vi "ProcessFCCurrentsSimple.vi"(9 "FC Data":waveform(dbl)[](array[waveform]), 10 "Bouncer Settings":T1 {"LE12C Voltage" format="%_4f"; "LE13C Voltage" format="%_4f"; "14C Voltage" format="%_4f"; "13C Voltage" format="%_4f"; "12C Voltage" format="%_4f"}, 11 "FC Offset":T2={"HE 12C Offset"=0.0, "HE 13CL Offset"=0.0, "HE 13CH Offset"=0.0, "LE FC Scale"=0, "HE C12 Scale"=0, "HE C13 Scale"=18} {"HE C13 Scale" items=["500 mA/V", "200 mA/V", "100 mA/V", "50 mA/V", "20 mA/V", "10 mA/V", "5 mA/V", "2 mA/V", "1 mA/V", "500 uA/V", "200 uA/V", "100 uA/V", "50 uA/V", "20 uA/V", "10 uA/V", "5 uA/V", "2 uA/V", "1 uA/V", "500 nA/V", "200 nA/V", "100 nA/V", "50 nA/V", "20 nA/V", "10 nA/V", "5 nA/V", "2 nA/V", "1 nA/V", "500 pA/V", "200 pA/V", "100 pA/V", "50 pA/V", "20 pA/V", "10 pA/V", "5 pA/V", "2 pA/V", "1 pA/V", ""]; "HE C12 Scale" items=["500 mA/V", "200 mA/V", "100 mA/V", "50 mA/V", "20 mA/V", "10 mA/V", "5 mA/V", "2 mA/V", "1 mA/V", "500 uA/V", "200 uA/V", "100 uA/V", "50 uA/V", "20 uA/V", "10 uA/V", "5 uA/V", "2 uA/V", "1 uA/V", "500 nA/V", "200 nA/V", "100 nA/V", "50 nA/V", "20 nA/V", "10 nA/V", "5 nA/V", "2 nA/V", "1 nA/V", "500 pA/V", "200 pA/V", "100 pA/V", "50 pA/V", "20 pA/V", "10 pA/V", "5 pA/V", "2 pA/V", "1 pA/V", ""]; "LE FC Scale" items=["500 mA/V", "200 mA/V", "100 mA/V", "50 mA/V", "20 mA/V", "10 mA/V", "5 mA/V", "2 mA/V", "1 mA/V", "500 uA/V", "200 uA/V", "100 uA/V", "50 uA/V", "20 uA/V", "10 uA/V", "5 uA/V", "2 uA/V", "1 uA/V", "500 nA/V", "200 nA/V", "100 nA/V", "50 nA/V", "20 nA/V", "10 nA/V", "5 nA/V", "2 nA/V", "1 nA/V", "500 pA/V", "200 pA/V", "100 pA/V", "50 pA/V", "20 pA/V", "10 pA/V", "5 pA/V", "2 pA/V", "1 pA/V", ""]}) -> (1 "Mean Currents":dbl[](array[numeric]), 2 "Output Waveforms":waveform(dbl)[](array[waveform]))   [LabVIEW 2011]
uses:
  FCOffset.ctl
  BouncerParameters.ctl
  <vilib>/Waveform/WDTOps.llb/WDT Get Waveform Subset DBL (LV80).vi
  <vilib>/Analysis/NI_AALBase.lvlib
panel:
  out "Raw":waveform(dbl)[](graph)
  out "HE 13CL":dbl
  out "HE 13CH":waveform(dbl)
  out "LE 13C":dbl
  out "HE 13CH":dbl
  out "LE 12C":dbl
  out "HE 12C":dbl
  out "Bouncer":waveform(dbl)(graph)={"t0"=timestamp(3415120333.4009705 s since 1904-01-01), "dt"=9.999999999999972e-06, "Y"=array[1000 elements], "attributes"=variant("NI_ChannelName"=variant(string "PXI1Slot2/ai0"), "NI_UnitDescription"=variant(string "Volts"))}
  out "LE 13C Cup":waveform(dbl)(graph)={"t0"=timestamp(3415120333.402178 s since 1904-01-01), "dt"=9.999999999999972e-06, "Y"=[0.8050097183722652, 0.24660166407635983, 0.028584441505206795, 0.009584422869030943, 0.009906457076575987, 0.00797425183471986, 0.00797425183471986, 0.007008149216862962, 0.012804764954733521, 0.01312679916455761, 0.010550525492349248, 0.010872559700577551, 0.009584422869030943, 0.01022849128434874, 0.01151662811771772, 0.010872559700577551, 0.010872559700577551, 0.010872559700577551, 0.01022849128434874, 0.009262388661713566, 0.004109841375562904, 0.009262388661713566, 0.01151662811771772, 0.01022849128434874, 0.019567483409006912, 0.01151662811771772, 0.010872559700577551, 0.009906457076575987, 0.009584422869030943, 0.01022849128434874, 0.013448833374609843, 0.01022849128434874, 0.009906457076575987, 0.010550525492349248, 0.00668611501136536, 0.010550525492349248, 0.01022849128434874, 0.01022849128434874, 0.009584422869030943, 0.013448833374609843], "attributes"=variant("NI_ChannelName"=variant(string "PXI1Slot2/ai3"), "NI_UnitDescription"=variant(string "Volts"))}
  out "LE 12C Cup":waveform(dbl)(graph)={"t0"=timestamp(3415120333.4013777 s since 1904-01-01), "dt"=9.999999999999972e-06, "Y"=[0.00668611501136536, 0.007008149216862962, 0.007652217628540168, 0.007330183422587883, 0.00861832024776164, 0.007330183422587883, 0.009262388661713566, 0.01312679916455761, 0.05338107720327494, 0.6781279926088322, 0.8175690797952145, 0.8223996035554544, 0.8240097781590372, 0.8233657083165931, 0.8249758829252316, 0.8230436733958766, 0.8243318130807649, 0.8236877432376466, 0.8243318130807649, 0.8243318130807649, 0.8233657083165931, 0.8278741972420289, 0.8236877432376466, 0.8240097781590372, 0.8227216384754971, 0.8246538480028296, 0.8246538480028296, 0.8246538480028296, 0.8249758829252316, 0.8252979178479707, 0.8214334987973474, 0.8236877432376466, 0.8246538480028296, 0.8246538480028296, 0.8227216384754971, 0.8236877432376466, 0.8243318130807649, 0.8217555337163797, 0.8240097781590372, 0.8243318130807649], "attributes"=variant("NI_ChannelName"=variant(string "PXI1Slot2/ai3"), "NI_UnitDescription"=variant(string "Volts"))}
  out "HE 13CL Cup":waveform(dbl)(graph)={"t0"=timestamp(3415120333.4017754 s since 1904-01-01), "dt"=9.999999999999972e-06, "Y"=[0.41889009921070675, 0.6410939957678486, 0.7270772818431984, 0.7261111773784867, 0.7270772818431984, 0.7293315256055366, 0.7267552470213039, 0.7286874559575331, 0.7306196649054364, 0.7254671077369653, 0.7283654211340178, 0.7302976300799747, 0.7277213514879598, 0.7261111773784867, 0.7306196649054364, 0.7341620480069433, 0.7293315256055366, 0.7302976300799747, 0.7319078042105287, 0.7331959435208164, 0.7280433863108267, 0.7331959435208164, 0.7290094907813727, 0.7299755952548376, 0.7309416997312226, 0.7344840828363023, 0.7293315256055366, 0.7299755952548376, 0.7267552470213039, 0.7338400131779094, 0.7219247247317432, 0.7225687943661443, 0.7280433863108267, 0.7280433863108267, 0.7309416997312226, 0.7290094907813727, 0.7328739086927573, 0.7277213514879598, 0.7161280980802982, 0.7286874559575331], "attributes"=variant("NI_ChannelName"=variant(string "PXI1Slot2/ai2"), "NI_UnitDescription"=variant(string "Volts"))}
  out "HE 12C Cup":waveform(dbl)(graph)={"t0"=timestamp(3415120333.400973 s since 1904-01-01), "dt"=9.999999999999972e-06, "Y"=[-0.00168677425192447, 0.003143738765882537, -0.002652876849375083, -0.00168677425192447, 0.0008894993512310448, -0.002652876849375083, 0.0005674651500443148, -0.000720671652438485, 0.0018556019561503992, 0.0018556019561503992, 0.0024996703605630385, 0.0015335677542840436, 0.002177636158243383, -0.0013647400523220184, 0.005397978191647298, 0.0018556019561503992, 0.0012115335526442733, 0.0015335677542840436, 0.016669175487689536, 0.2607711773435167, 0.6375516136789285, 0.6369075442122739, 0.6423821347186465, 0.6456024821175347, 0.6449584126352536, 0.6423821347186465, 0.6456024821175347, 0.6427041694571275, 0.639805856822051, 0.6427041694571275, 0.6388397526159826, 0.6449584126352536, 0.6423821347186465, 0.6443143431542244, 0.6452804473762376, 0.6401278915580318, 0.6410939957678486, 0.6468906210858548, 0.6446363778945825, 0.6433482389350278], "attributes"=variant("NI_ChannelName"=variant(string "PXI1Slot2/ai1"), "NI_UnitDescription"=variant(string "Volts"))}
  # "ms"
  # "us"
  # "kV"
  # "ms"
  # "us"
  # "kV"
  # "ms"
  # "us"
  # "kV"
  # "ms"
  # "us"
  # "kV"
  # "ms"
  # "us"
  # "kV"
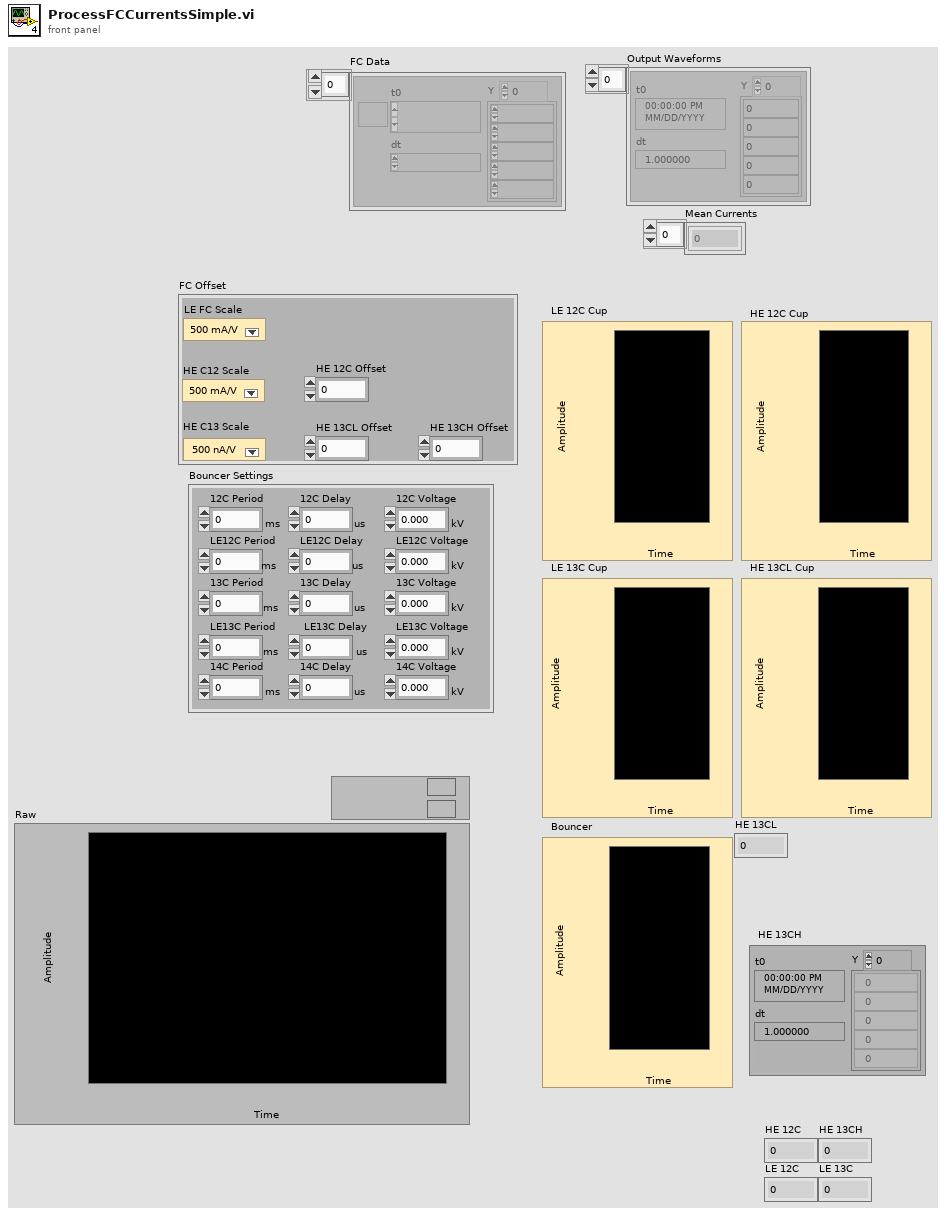
[diagram p1: front panel]
types:
  T1 = typedef "BouncerParameters.ctl" = cluster{"12C Period":dbl, "12C Delay":dbl, "12C Voltage":dbl, "13C Period":dbl, "13C Delay":dbl, "13C Voltage":dbl, "14C Period":dbl, "14C Delay":dbl, "14C Voltage":dbl, "LE13C Period":dbl, "LE13C Delay":dbl, "LE13C Voltage":dbl, "LE12C Period":dbl, "LE12C Delay":dbl, "LE12C Voltage":dbl}
  T2 = typedef "FCOffset.ctl" = cluster{"HE 12C Offset":dbl, "HE 13CL Offset":dbl, "HE 13CH Offset":dbl, "LE FC Scale":u16, "HE C12 Scale":u16, "HE C13 Scale":u16}
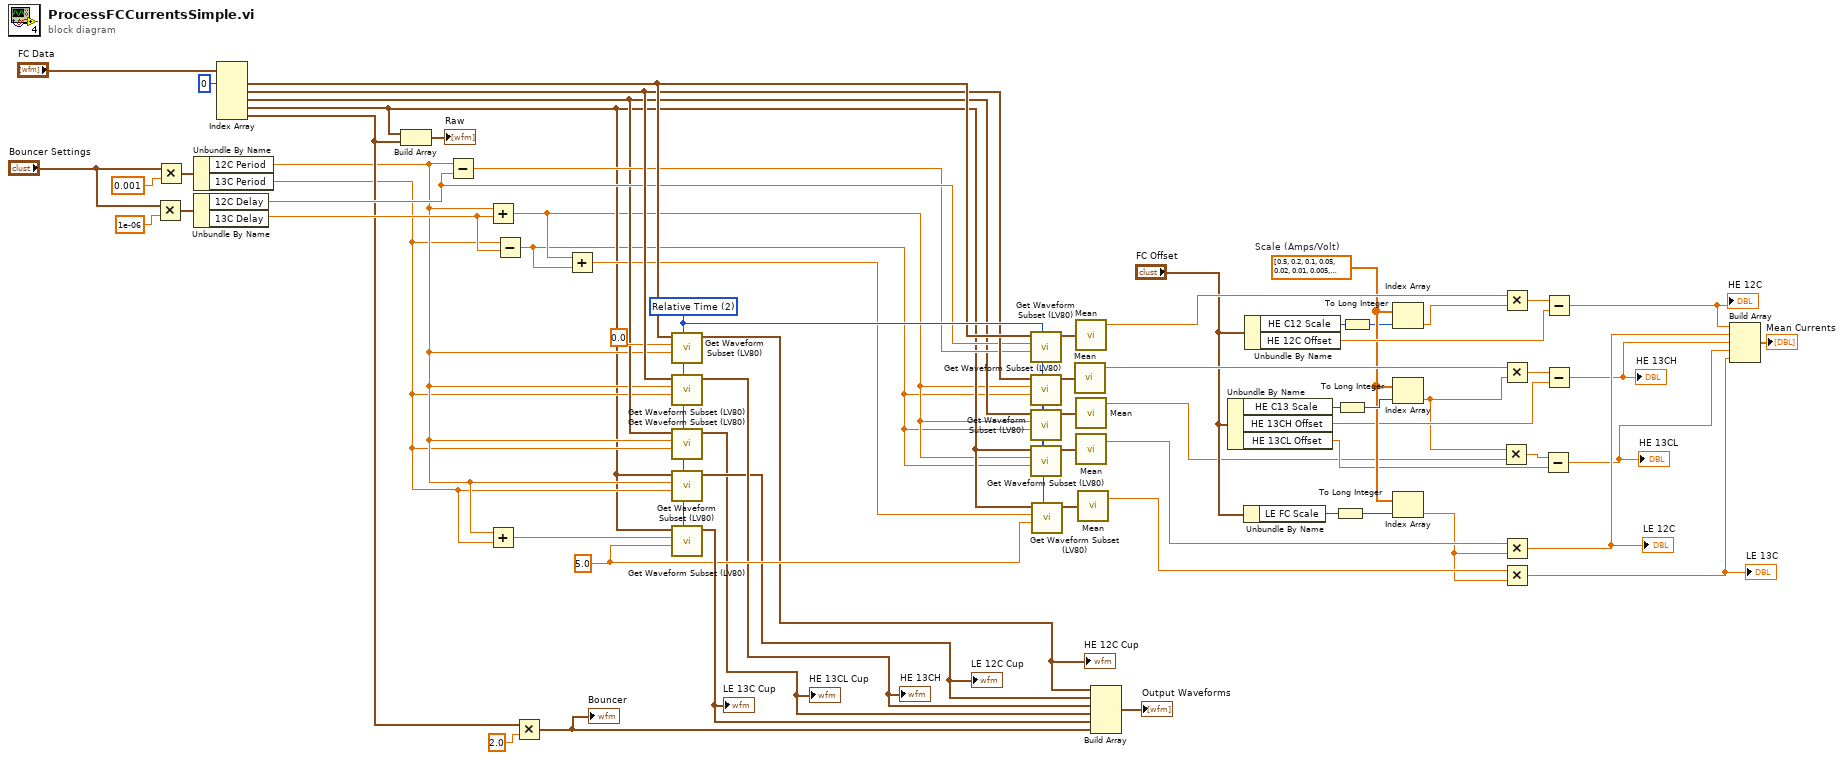
[diagram p0: block diagram]
diagram:
  w17 = 5.0 ("duration")
  w38 = dbl[] [0.5, 0.2, 0.1, 0.05, 0.02, 0.01, 0.005, 0.002, 0.001, 0.0005, 0.0002, 0.0001, 5e-05, 2e-05, 1e-05, 5e-06, 2e-06, 1e-06, 5e-07, 2e-07, 1e-07, 5e-08, 2e-08, 1e-08, 5e-09, 2e-09, 1e-09, 5e-10, 2e-10, 1e-10, 5e-11, 2e-11, 1e-11, 5e-12, 2e-12, 1e-12]  # Scale (Amps/Volt)
  w42 = u16 2 items=["Samples", "Absolute Time", "Relative Time"] ("start/duration format")
  n1 = Multiply(x="Bouncer Settings", y=1e-06) -> (x*y=w62:T1)
  n2 = Multiply(x="Bouncer Settings", y=0.001) -> (x*y=w64:T1)
  n3 = Unbundle By Name(w64) -> ("12C Period"=w21:dbl, "13C Period"=w20:dbl)
  n4 = Unbundle By Name(w62) -> ("12C Delay"=w32:dbl, "13C Delay"=w30:dbl)
  n5 = Index Array(array="FC Data", index #1=0 ("index")) -> (element #1=w36:waveform(dbl), element #2=w35:waveform(dbl), element #3=w29:waveform(dbl), element #4=w5:waveform(dbl), element #5=w25:waveform(dbl))  [unwired: 4 in]
  n6 = Build Array(w5, w25) -> (→"Raw":waveform(dbl)[])
  n7 = Subtract(x=w21, y=w32) -> (x-y=w31:dbl)
  n8 = Add(x=w21, y=w30) -> (x+y=w4:dbl)
  n9 = Add(x=w21, y=w20) -> (x+y=w19:dbl)
  n10 = Subtract(x=w20, y=w30) -> (x-y=w3:dbl)
  n11 = Multiply(x=w25, y=2.0) -> (x*y=w34:waveform(dbl))
  "Bouncer" <- w34
  n12 = Add(x=w4, y=w3) -> (x+y=w18:dbl)
  n13 = call-poly <vilib>:"Get Waveform Subset (LV80).vi"("start/duration format"=w42, "duration"=w21, "start samples/time"=0.0, "waveform in"=w36) -> ("waveform out"=w6:waveform(dbl))  [unwired: 1 in, 4 out]
  "HE 12C Cup" <- w6
  n14 = call-poly <vilib>:"Get Waveform Subset (LV80).vi"("start/duration format"=w42, "duration"=w20, "start samples/time"=w21, "waveform in"=w35) -> ("waveform out"=w8:waveform(dbl))  [unwired: 1 in, 4 out]
  "HE 13CH" <- w8
  n15 = call-poly <vilib>:"Get Waveform Subset (LV80).vi"("start/duration format"=w42, "duration"=w20, "start samples/time"=w21, "waveform in"=w29) -> ("waveform out"=w2:waveform(dbl))  [unwired: 1 in, 4 out]
  "HE 13CL Cup" <- w2
  n16 = call-poly <vilib>:"Get Waveform Subset (LV80).vi"("start/duration format"=w42, "duration"=w20, "start samples/time"=w21, "waveform in"=w5) -> ("waveform out"=w7:waveform(dbl))  [unwired: 1 in, 4 out]
  "LE 12C Cup" <- w7
  n17 = call-poly <vilib>:"Get Waveform Subset (LV80).vi"("start/duration format"=w42, "duration"=w17, "start samples/time"=w19, "waveform in"=w5) -> ("waveform out"=w24:waveform(dbl))  [unwired: 1 in, 4 out]
  "LE 13C Cup" <- w24
  n18 = call-poly <vilib>:"Get Waveform Subset (LV80).vi"("start/duration format"=w42, "duration"=w31, "start samples/time"=w32, "waveform in"=w36) -> ("waveform out"=w60:waveform(dbl))  [unwired: 1 in, 4 out]
  n19 = call-poly <vilib>:"Get Waveform Subset (LV80).vi"("start/duration format"=w42, "duration"=w3, "start samples/time"=w4, "waveform in"=w35) -> ("waveform out"=w58:waveform(dbl))  [unwired: 1 in, 4 out]
  n20 = call-poly <vilib>:"Get Waveform Subset (LV80).vi"("start/duration format"=w42, "duration"=w3, "start samples/time"=w4, "waveform in"=w29) -> ("waveform out"=w41:waveform(dbl))  [unwired: 1 in, 4 out]
  n21 = call-poly <vilib>:"Get Waveform Subset (LV80).vi"("start/duration format"=w42, "duration"=w3, "start samples/time"=w4, "waveform in"=w5) -> ("waveform out"=w57:waveform(dbl))  [unwired: 1 in, 4 out]
  n22 = call-poly <vilib>:"Get Waveform Subset (LV80).vi"("start/duration format"=w42, "duration"=w17, "start samples/time"=w18, "waveform in"=w5) -> ("waveform out"=w59:waveform(dbl))  [unwired: 1 in, 4 out]
  n23 = call <vilib>:"Mean.vi"("X"=w58) -> ("mean"=w55:dbl)  [unwired: 1 out]
  n24 = call <vilib>:"Mean.vi"("X"=w60) -> ("mean"=w56:dbl)  [unwired: 1 out]
  n25 = call <vilib>:"Mean.vi"("X"=w41) -> ("mean"=w1:dbl)  [unwired: 1 out]
  n26 = call <vilib>:"Mean.vi"("X"=w57) -> ("mean"=w23:dbl)  [unwired: 1 out]
  n27 = call <vilib>:"Mean.vi"("X"=w59) -> ("mean"=w22:dbl)  [unwired: 1 out]
  n28 = Build Array(w6, w7, w8, w2, w24, w34) -> (→"Output Waveforms":waveform(dbl)[])
  n29 = Unbundle By Name("FC Offset") -> ("HE C13 Scale"=w54:u16, "HE 13CH Offset"=w14:dbl, "HE 13CL Offset"=w10:dbl)
  n30 = Unbundle By Name("FC Offset") -> ("LE FC Scale"=w13:u16)
  n31 = Unbundle By Name("FC Offset") -> ("HE C12 Scale"=w16:u16, "HE 12C Offset"=w51:dbl)
  n32 = To Long Integer(number=w13) -> (32bit integer=w12:i32)
  n33 = To Long Integer(number=w54) -> (32bit integer=w50:i32)
  n34 = To Long Integer(number=w16) -> (32bit integer=w15:i32)
  n35 = Index Array(array=w38, index=w15) -> (element=w28:dbl)
  n36 = Index Array(array=w38, index=w50) -> (element=w9:dbl)
  n37 = Index Array(array=w38, index=w12) -> (element=w11:dbl)
  n38 = Multiply(x=w9, y=w1) -> (x*y=w40:dbl)
  n39 = Multiply(x=w56, y=w28) -> (x*y=w53:dbl)
  n40 = Multiply(x=w55, y=w9) -> (x*y=w52:dbl)
  n41 = Multiply(x=w23, y=w11) -> (x*y=w46:dbl)
  "LE 12C" <- w46
  n42 = Multiply(x=w22, y=w11) -> (x*y=w44:dbl)
  "LE 13C" <- w44
  n43 = Subtract(x=w40, y=w10) -> (x-y=w39:dbl)
  "HE 13CL" <- w39
  n44 = Subtract(x=w53, y=w51) -> (x-y=w47:dbl)
  "HE 12C" <- w47
  n45 = Subtract(x=w52, y=w14) -> (x-y=w45:dbl)
  "HE 13CH" <- w45
  n46 = Build Array(w47, w46, w45, w39, w44) -> (→"Mean Currents":dbl[])
